vi "CAN_Init-8.6.vi"(0 "CAN卡类型":u32(ring)=4 items=["PCI5121"=1, "PCI9810"=2, "USBCAN1"=3, "USBCAN2"=4, "PCI9820"=5, "PCI5110"=7, "CANLite(mini)"=8, "ISA9620"=9, "ISA5420"=10, "PC104CAN"=11, "DNP9810"=13, "PCI9840B"=14, "PC104C2"=15, "PCI9820I"=16, "pec9920"=18, "USBCAN_E_U"=20, "USBCAN_2E_U"=21], 1 "设备索引号":u16(ring) items=["0", "1", "2", "3", "4", "5", "6", "7", "8", "9", "10", "11", "12", "13", "14", "15", ""], 2 "CAN端口":u16(ring) items=["0", "1"], 3 "波特率":T5(ring)=enum."500Kbps", 4 "操作类型":enum16{"初始化CAN", "关闭CAN"}(ring), 5 "error in (no error)":errorcluster caption="错误输入（无错误）", 6 "滤波方式":u8(ring)=1 items=["Dual Filter", "Single Filter"], 7 "Accept Code":u32 format="%08x", 8 "簇":T3={"打开CAN"=TRUE, "初始化CAN"=TRUE, "开始CAN"=TRUE, "重启"=TRUE, "关闭CAN"=TRUE}, 9 "Mask Code":u32=4294967295 format="%08x", 10 "工作方式":u8(ring) items=["Normal", "Listen Only"], 11 "E-U_baud":u32(ring)=393223 items=["0x060003--1000Kbps"=393219, "0x060004--800Kbps"=393220, "0x060007--500Kbps"=393223, "0x1C0008--250Kbps"=1835016, "0x1C0011--125Kbps"=1835025, "0x160023--100Kbps"=1441827, "0x1C002C--50Kbps"=1835052, "0x1600B3--20Kbps"=1441971, "0x1C00E0--10Kbps"=1835232, "0x1C01C1--5Kbps"=1835457], 12 "是否滤波":bool, 13 "滤波选择":T2={"fiter_mode"=1, "fiter_endid"=0, "fiter_startid"=0} {"fiter_mode" items=["标准帧滤波", "扩展帧滤波", "禁能滤波"]}) -> (14 "CAN 操作结果":bool=TRUE, 18 "真":bool, 19 "error out":errorcluster caption="错误输出")   [LabVIEW 2013]
uses:
  data/ControlCAN.dll
panel:
  out "跳过":bool
  out "数值":u32
  out "VCI_CAN_STATUS 2":T1
  out "ret_ok":bool=TRUE
  out "VCI_FILTER_RECORD":cluster{"ExtFrame":u32, "Start":u32, "End":u32}
  in  "e-u-baud":cluster{"数值":u32}
  in  "VCI_INIT_CONFIG":T4={"AccCode"=0, "AccMask"=4294967295, "Reserved"=0, "Filter"=0, "Timing0"=0, "Timing1"=28, "Mode"=0}
  in  "DeviceType 5":u16(ring)=1 items=["PCI5121"=1, "PCI9810"=2, "USBCAN1"=3, "USBCAN2"=4, "PCI9820"=5, "CAN232"=6, "PCI5110"=7, "CANLite(mini)"=8, "ISA9620"=9, "ISA5420"=10, "PC104CAN"=11, "CANETE"=12, "DNP9810"=13]
  in  "CAN Channel 3":u16(ring) items=["0", "1"]
  in  "DeviceType 4":u16(ring)=1 items=["PCI5121"=1, "PCI9810"=2, "USBCAN1"=3, "USBCAN2"=4, "PCI9820"=5, "CAN232"=6, "PCI5110"=7, "CANLite(mini)"=8, "ISA9620"=9, "ISA5420"=10, "PC104CAN"=11, "CANETE"=12, "DNP9810"=13]
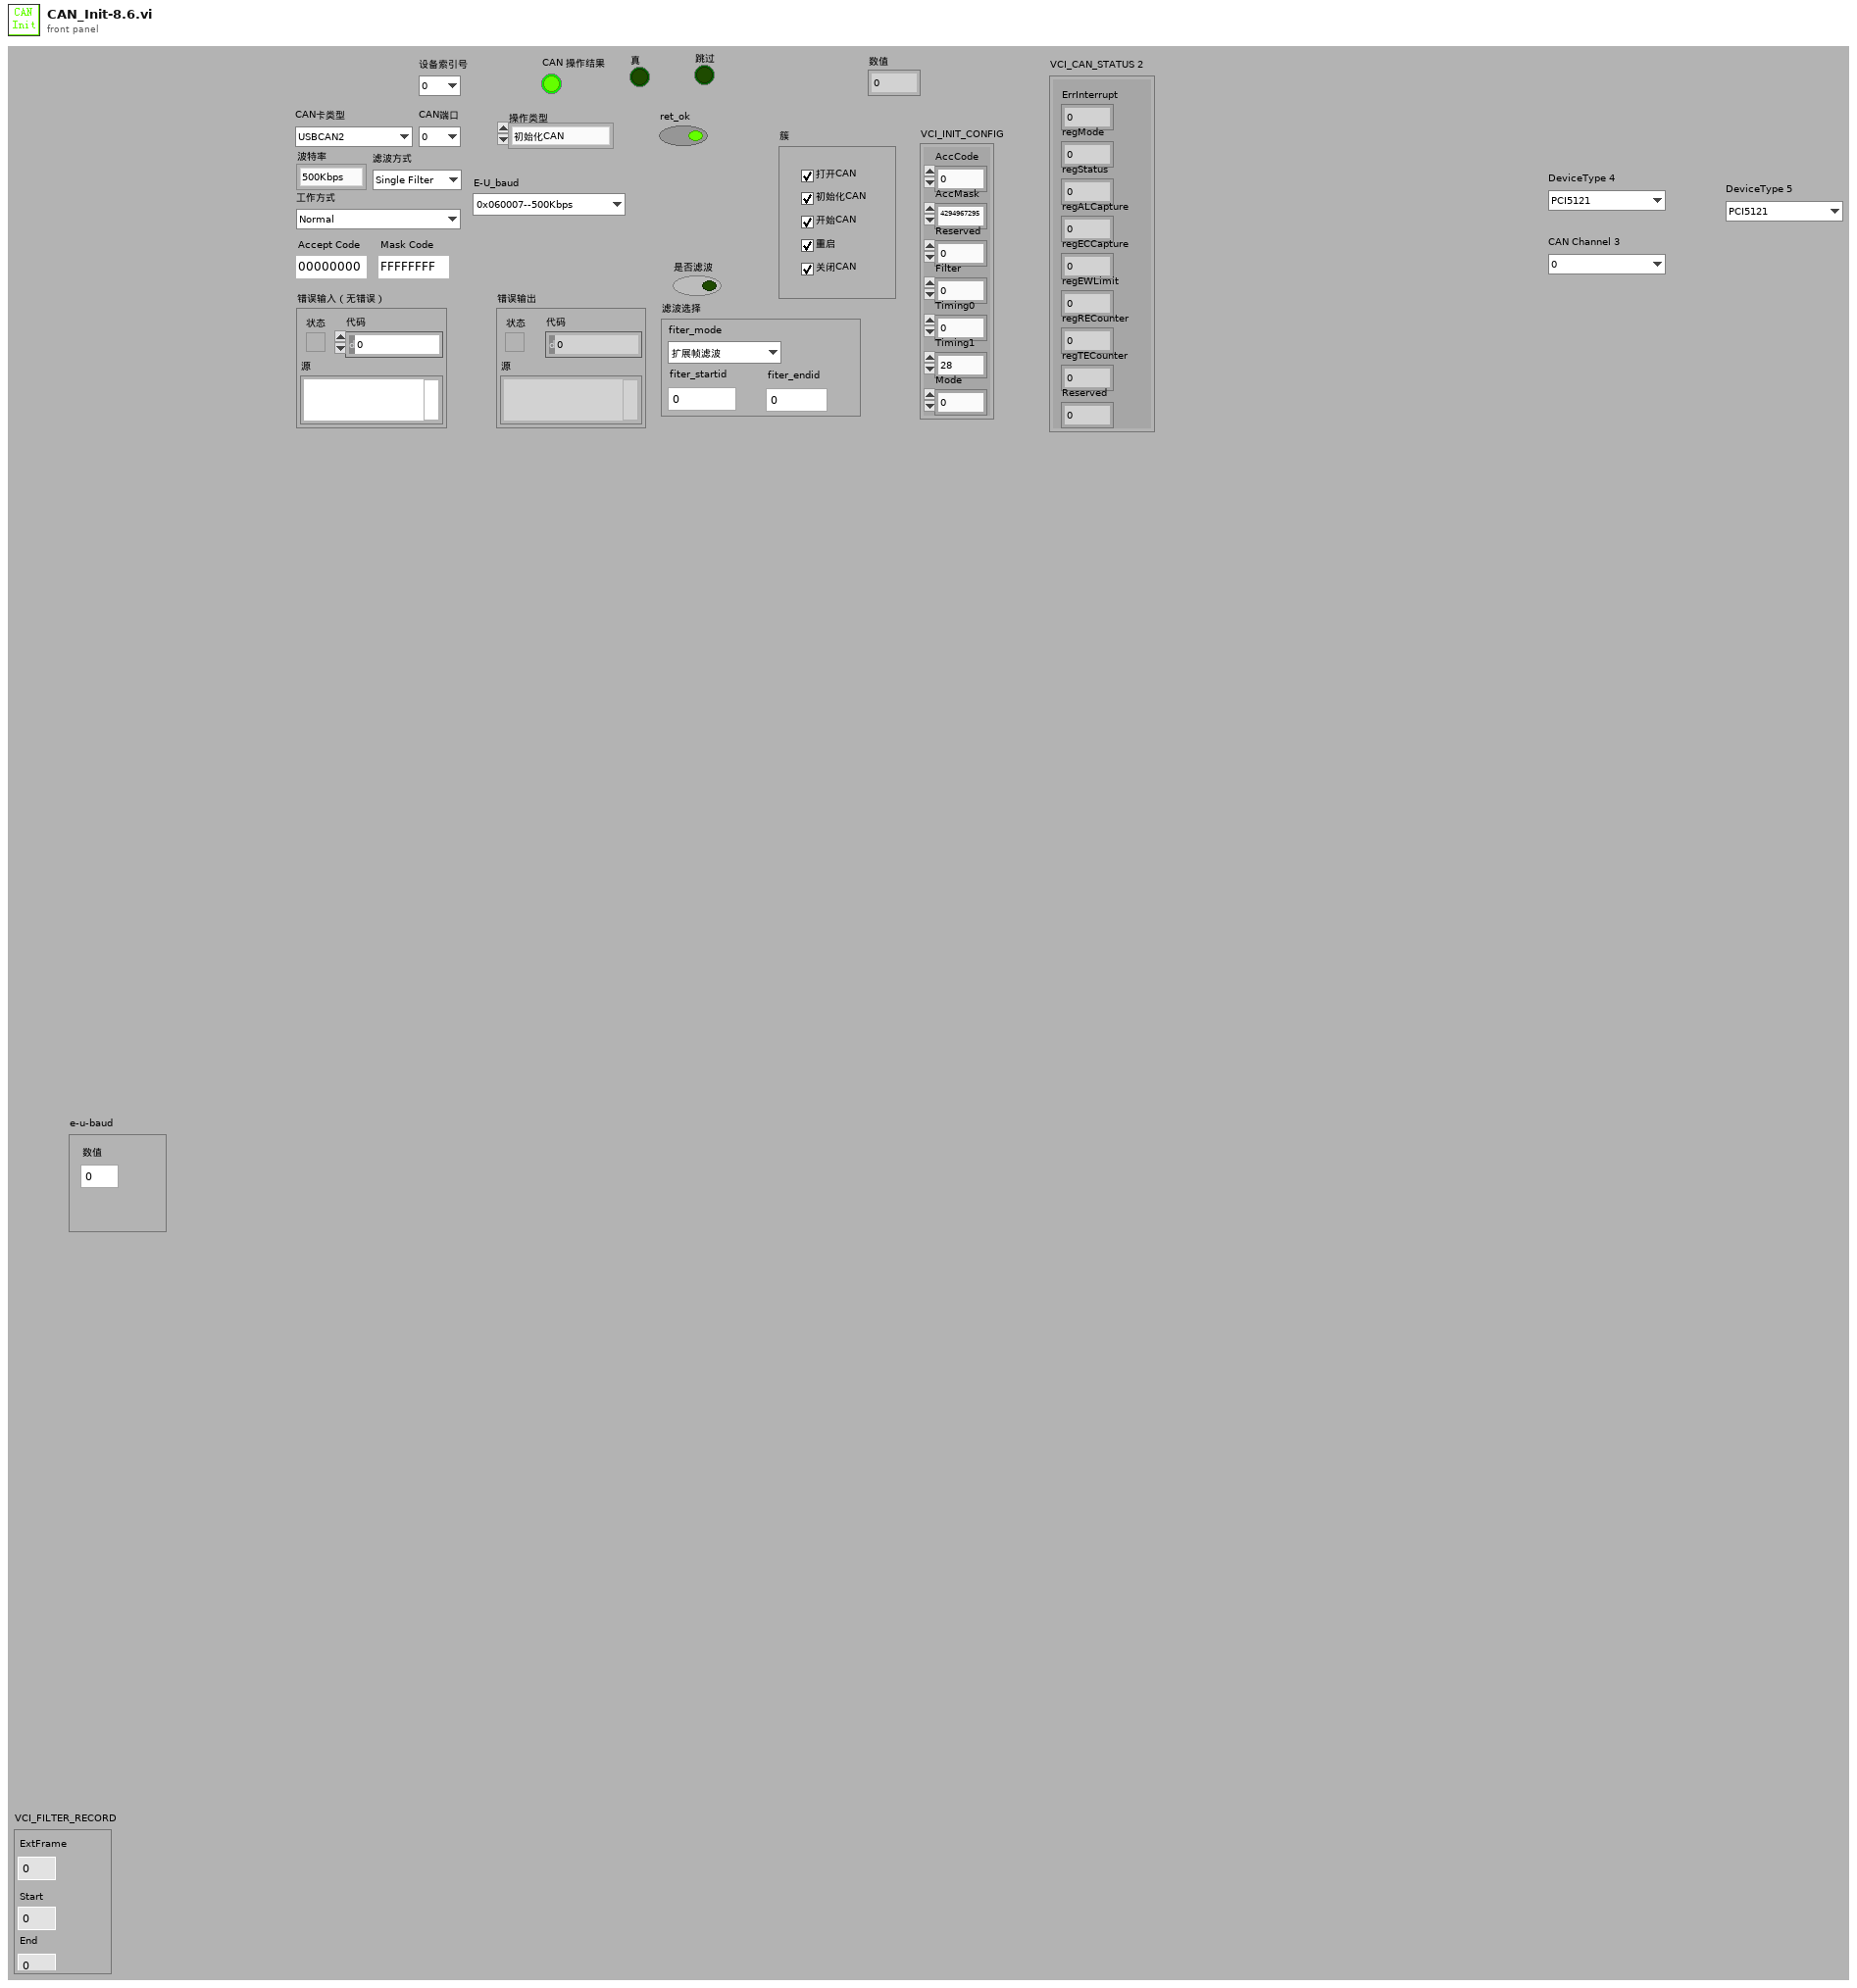
[diagram p1: front panel]
types:
  T1 = cluster{"ErrInterrupt":u8, "regMode":u8, "regStatus":u8, "regALCapture":u8, "regECCapture":u8, "regEWLimit":u8, "regRECounter":u8, "regTECounter":u8, "Reserved":u32}
  T2 = cluster{"fiter_mode":u32, "fiter_endid":u32, "fiter_startid":u32}
  T3 = cluster{"打开CAN":bool, "初始化CAN":bool, "开始CAN":bool, "重启":bool, "关闭CAN":bool}
  T4 = cluster{"AccCode":u32, "AccMask":u32, "Reserved":u32, "Filter":u8, "Timing0":u8, "Timing1":u8, "Mode":u8}
  T5 = enum16{"5Kbps", "10Kbps", "20Kbps", "40Kbps", "50Kbps", "80Kbps", "100Kbps", "125Kbps", "200Kbps", "250Kbps", "400Kbps", "500Kbps", "666Kbps", "800Kbps", "1000Kbps"}
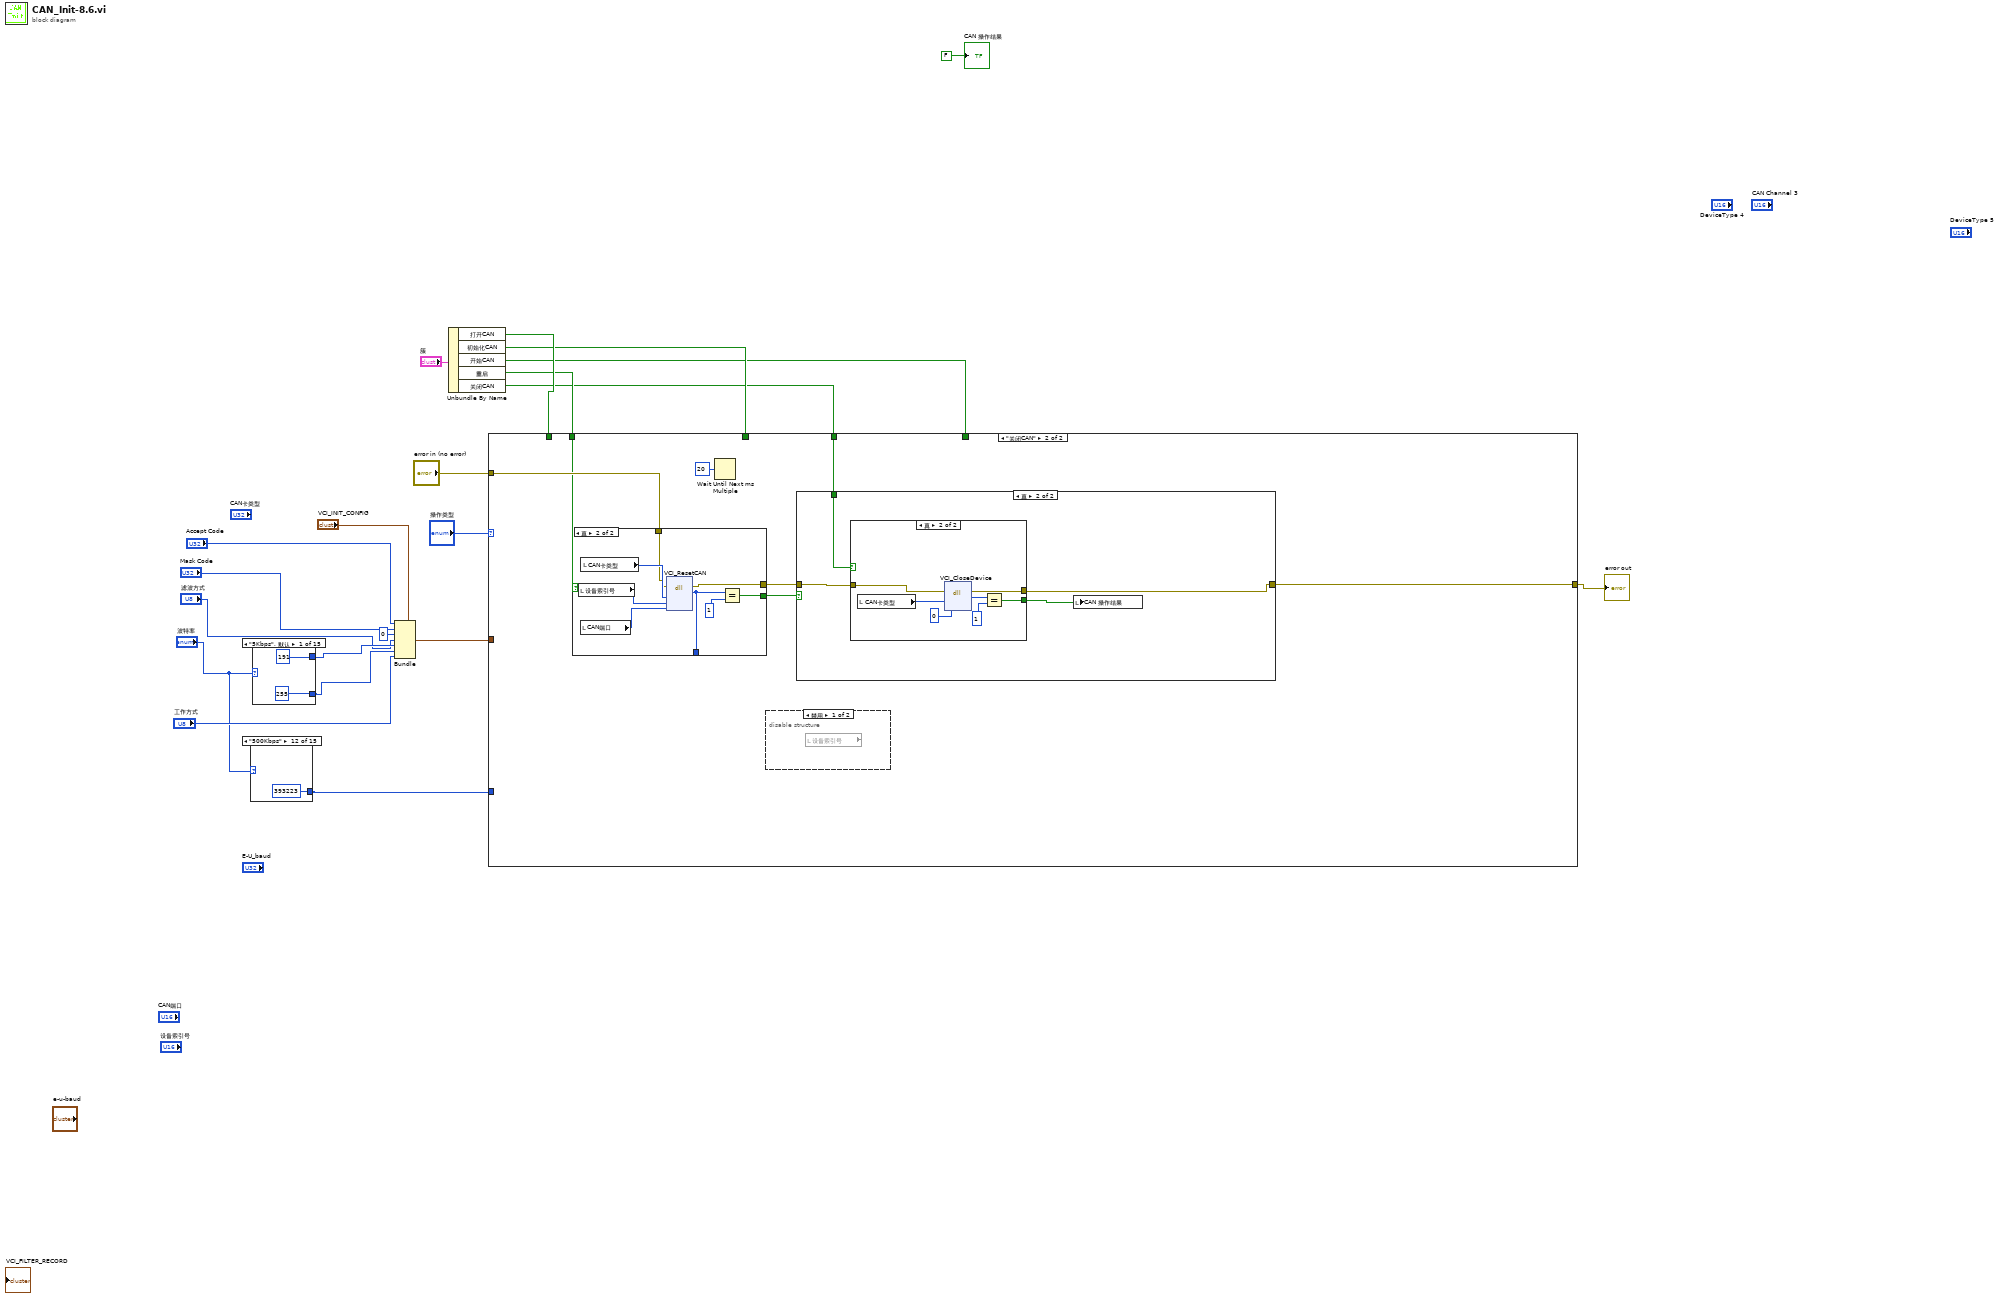
[diagram p0: block diagram]
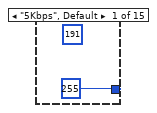
[diagram p2: hidden frame]
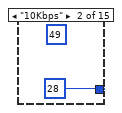
[diagram p3: hidden frame]
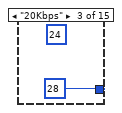
[diagram p4: hidden frame]
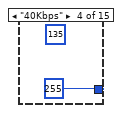
[diagram p5: hidden frame]
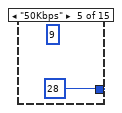
[diagram p6: hidden frame]
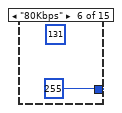
[diagram p7: hidden frame]
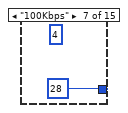
[diagram p8: hidden frame]
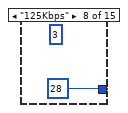
[diagram p9: hidden frame]
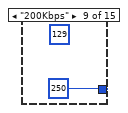
[diagram p10: hidden frame]
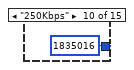
[diagram p11: hidden frame]
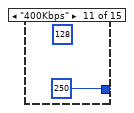
[diagram p12: hidden frame]
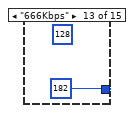
[diagram p13: hidden frame]
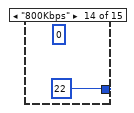
[diagram p14: hidden frame]
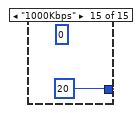
[diagram p15: hidden frame]
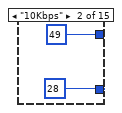
[diagram p16: hidden frame]
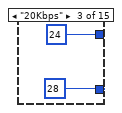
[diagram p17: hidden frame]
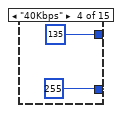
[diagram p18: hidden frame]
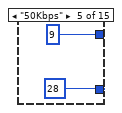
[diagram p19: hidden frame]
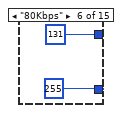
[diagram p20: hidden frame]
diagram:
  n1 = case shown="\"500Kbps\"" "波特率" {
    tunnel: [255 28 28 255 28 255 28 28 250 1835016 250 393223 182 22 20] -> w1
    frame "5Kbps", Default {
      (unwired) 191
    }
    frame "10Kbps" {
      (unwired) 49
    }
    frame "20Kbps" {
      (unwired) 24
    }
    frame "40Kbps" {
      (unwired) 135
    }
    frame "50Kbps" {
      (unwired) 9
    }
    frame "80Kbps" {
      (unwired) 131
    }
    frame "100Kbps" {
      (unwired) 4
    }
    frame "125Kbps" {
      (unwired) 3
    }
    frame "200Kbps" {
      (unwired) 129
    }
    frame "250Kbps" {
    }
    frame "400Kbps" {
      (unwired) 128
    }
    frame "500Kbps" {
    }
    frame "666Kbps" {
      (unwired) 128
    }
    frame "800Kbps" {
      (unwired) 0
    }
    frame "1000Kbps" {
      (unwired) 0
    }
  }
  n2 = case shown="\"5Kbps\", 默认" "波特率" {
    tunnel: [191 49 24 135 9 131 4 3 129 1 128 0 128 0 0] -> w20
    tunnel: [255 28 28 255 28 255 28 28 250 28 250 28 182 22 20] -> w19
    frame "5Kbps", Default {
    }
    frame "10Kbps" {
    }
    frame "20Kbps" {
    }
    frame "40Kbps" {
    }
    frame "50Kbps" {
    }
    frame "80Kbps" {
    }
    frame "100Kbps" {
    }
    frame "125Kbps" {
    }
    frame "200Kbps" {
    }
    frame "250Kbps" {
    }
    frame "400Kbps" {
    }
    frame "500Kbps" {
    }
    frame "666Kbps" {
    }
    frame "800Kbps" {
    }
    frame "1000Kbps" {
    }
  }
  n3 = Bundle(cluster="VCI_INIT_CONFIG", "AccCode"="Accept Code", "AccMask"="Mask Code", "Reserved"=u32 0, "Filter"="滤波方式", "Timing0"=w20, "Timing1"=w19, "Mode"="工作方式") -> (w16:T4)
  n4 = Unbundle By Name("簇") -> ("打开CAN"=w9:bool, "初始化CAN"=w8:bool, "开始CAN"=w7:bool, "重启"=w6:bool, "关闭CAN"=w5:bool)
  n5 = case shown="\"关闭CAN\"" "操作类型" {
    tunnel: w16 -> [w73 _]
    tunnel: "error in (no error)" -> [w72 w242]
    tunnel: [w71 w240] -> w4
    tunnel: w9 -> [w70 _]
    tunnel: w8 -> [w69 _]
    tunnel: w7 -> [w68 _]
    tunnel: w6 -> [_ w239]
    tunnel: w5 -> [_ w238]
    tunnel: w1 -> [w67 _]
    frame "初始化CAN", Default {
      n6 = stacked-sequence {
        seq-local: [w74 _] -> [_ w84]
        tunnel: w73 -> [_ w90]
        tunnel: w72 -> [_ w89]
        tunnel: [_ w88] -> w71
        tunnel: w70 -> [_ w87]
        tunnel: w69 -> [_ w86]
        tunnel: w68 -> [_ w85]
        tunnel: w67 -> [_ w83]
        frame #0 {
          n7 = disable-structure shown="禁用" {
            disable-tunnel: [w75 _] -> w74
            frame Disabled {
              n8 = local read "CAN卡类型"() -> (w81:u32)
              n9 = local read "CAN端口"() -> (w80:u16)
              n10 = dll-call lib="PTH1Fabs EDelan\t上位机BMS_Monitor - 91版_1dataControlCAN.dll" fn="VCI_ReadCANStatus"("DeviceType"=w81, "DeviceInd"=u32 0, "CANInd"=w80) -> ("返回类型"=→"数值":u32, "VCI_CAN_STATUS 2"=w78:T1)  [unwired: 5 in, 4 out]
              "VCI_CAN_STATUS 2" <- w78
              n11 = Unbundle By Name(w78) -> ("regStatus"=w77:u8)
              n12 = Equal?(x=w77, y=u8 18) -> (x = y?=w75:bool)
            }
            frame Enabled {
            }
          }
          "跳过" <- w74
        }
        frame #1 {
          n13 = case shown="假" w84 {
            tunnel: w90 -> [w99 _]
            tunnel: w89 -> [w98 _]
            tunnel: [w96 _] -> w88
            tunnel: w87 -> [w94 _]
            tunnel: w86 -> [w93 _]
            tunnel: w85 -> [w92 _]
            tunnel: w83 -> [w91 _]
            frame False {
              n14 = local read "CAN卡类型"() -> (w95:u32)
              n15 = case shown="真" w94 {
                tunnel: [TRUE w111] -> w101
                tunnel: [w103 w107] -> w100
                tunnel: w98 -> [w105 w110]
                tunnel: [w105 w109] -> w97
                tunnel: [u32 1 ("返回类型") w108] -> _
                tunnel: w95 -> [w103 w107]
                frame False {
                }
                frame True {
                  w106 = 0
                  n16 = dll-call lib="PTH1Fabs EDelan\t上位机BMS_Monitor - 91版_1dataControlCAN.dll" fn="VCI_OpenDevice"(error in=w110, "DevType"=w107, "DevIndex"=w106, "Reserved"=w106) -> (error out=w109:errorcluster, "返回类型"=w108:u32)  [unwired: 4 in, 2 out]
                  n17 = Equal?(x=w108, y=u32 1) -> (x = y?=w111:bool)
                }
              }
              n18 = case shown="真" w101 {
                tunnel: w100 -> [_ w131]
                tunnel: w99 -> [_ w128]
                tunnel: w97 -> [w118 w127]
                tunnel: [w118 w130] -> w96
                tunnel: w93 -> [_ w124]
                tunnel: w92 -> [_ w129]
                tunnel: w91 -> [_ w123]
                frame False {
                  n19 = global read "中英文全局-8.6.vi" "英文?"() -> (w113:bool)
                  n20 = case shown="真" w113 {
                    tunnel: ["Error opening CAN" ("消息") "打开CAN错误" ("消息")] -> w115
                    tunnel: ["Yes" ("按钮名称（“确定”）") "确定" ("按钮名称（“确定”）")] -> w114
                    frame True {
                    }
                    frame False {
                    }
                  }
                  n21 = local write "CAN 操作结果"(FALSE ("初始化结果")) -> ()
                  n22 = One Button Dialog(message=w115, button name ("OK")=w114) -> (true=w116:bool)
                  n23 = local write "真"(w116) -> ()
                }
                frame True {
                  n24 = stacked-sequence {
                    seq-local: [w134 _ _ _] -> [_ w142 _ w193]
                    tunnel: w128 -> [_ _ w171 _]
                    tunnel: [_ _ w170 _] -> _
                    tunnel: w127 -> [_ w141 w169 _]
                    tunnel: [_ _ w168 _] -> w126
                    tunnel: [_ _ w167 _] -> w125
                    tunnel: w124 -> [_ _ w165 _]
                    tunnel: w123 -> [_ w140 _ _]
                    frame #0 {
                      w137 = u32 21 items=["PCI5121"=1, "PCI9810"=2, "USBCAN1"=3, "USBCAN2"=4, "PCI9820"=5, "PCI5110"=7, "CANLite(mini)"=8, "ISA9620"=9, "ISA5420"=10, "PC104CAN"=11, "DNP9810"=13, "PCI9840B"=14, "PC104C2"=15, "PCI9820I"=16, "pec9920"=18, "USBCAN_E_U"=20, "USBCAN_2E_U"=21, ""=0] ("DeviceType")
                      w139 = u32 20 items=["PCI5121"=1, "PCI9810"=2, "USBCAN1"=3, "USBCAN2"=4, "PCI9820"=5, "PCI5110"=7, "CANLite(mini)"=8, "ISA9620"=9, "ISA5420"=10, "PC104CAN"=11, "DNP9810"=13, "PCI9840B"=14, "PC104C2"=15, "PCI9820I"=16, "pec9920"=18, "USBCAN_E_U"=20, "USBCAN_2E_U"=21, ""=0] ("DeviceType")
                      # "判断是不是USB_U_E设备"
                      n25 = local read "CAN卡类型"() -> (w138:u32)
                      n26 = Equal?(x=w138, y=w139) -> (x = y?=w136:bool)
                      n27 = Equal?(x=w138, y=w137) -> (x = y?=w135:bool)
                      n28 = Or(x=w136, y=w135) -> (x .or. y?=w134:bool)
                      n29 = Wait Until Next ms Multiple(millisecond multiple=u32 10 ("毫秒倍数")) -> ()  [unwired: 1 out]
                      "ret_ok" <- TRUE ("ret_ok")
                    }
                    frame #1 {
                      n30 = case shown="真" w142 {
                        tunnel: w141 -> [w143 w148]
                        tunnel: [w143 w147] -> _
                        tunnel: w140 -> [_ w144]
                        frame False {
                          # "不是 -U-E 设备，不做处理"
                        }
                        frame True {
                          # "设置波特率"
                          # "USB-E-U初始化"
                          n31 = local read "CAN卡类型"() -> (w152:u32)
                          n32 = local read "设备索引号"() -> (w151:u16)
                          n33 = local read "CAN端口"() -> (w150:u16)
                          n34 = Bundle(w144) -> (w149:cluster{i32})  [unwired: 1 in]
                          n35 = dll-call lib="PTH1Fabs EDelan\t上位机BMS_Monitor - 91版_1dataControlCAN.dll" fn="VCI_SetReference"(error in=w148, "DevType"=w152, "DevIndex"=w151, "CANInd"=w150, "RefType"=u32 0, "pData"=w149) -> (error out=w147:errorcluster, "返回类型"=w154:u32)  [unwired: 5 in, 3 out]
                          n36 = Wait Until Next ms Multiple(millisecond multiple=u32 10 ("毫秒倍数")) -> ()  [unwired: 1 out]
                          n37 = Equal?(x=w154, y=u32 1) -> (x = y?=w145:bool)
                          n38 = local write "ret_ok"(w145) -> ()
                          n39 = case shown="假" w145 {
                            frame False {
                              n40 = global read "中英文全局-8.6.vi" "英文?"() -> (w156:bool)
                              n41 = case shown="真" w156 {
                                tunnel: ["Set the baud rate error, open the equipment failure" ("消息") "设置波特率错误，打开设备失败" ("消息")] -> w159
                                tunnel: ["Yes" ("按钮名称（“确定”）") "Yes" ("按钮名称（“确定”）")] -> w158
                                frame True {
                                }
                                frame False {
                                }
                              }
                              n42 = One Button Dialog(message=w159, button name ("OK")=w158) -> (true=w157:bool)
                              n43 = local write "真"(w157) -> ()
                            }
                            frame True {
                            }
                          }
                        }
                      }
                    }
                    frame #2 {
                      n44 = local read "ret_ok"() -> (w164:bool)
                      n45 = And(x=w164, y=w165) -> (x .and. y?=w166:bool)
                      n46 = case shown="真" w166 {
                        tunnel: w171 -> [_ w178]
                        tunnel: [_ w177] -> w170
                        tunnel: w169 -> [w172 w176]
                        tunnel: [w172 w175] -> w168
                        tunnel: [_ w174] -> w167
                        tunnel: w164 -> [_ _]
                        frame False {
                        }
                        frame True {
                          n47 = local read "CAN卡类型"() -> (w181:u32)
                          n48 = local read "设备索引号"() -> (w180:u16)
                          n49 = local read "CAN端口"() -> (w179:u16)
                          n50 = dll-call lib="PTH1Fabs EDelan\t上位机BMS_Monitor - 91版_1dataControlCAN.dll" fn="VCI_InitCAN"(error in=w176, "DeviceType"=w181, "DeviceInd"=w180, "CANInd"=w179, "pInitConfig"=w178) -> (error out=w175:errorcluster, "返回类型"=w177:u32)  [unwired: 4 in, 3 out]
                          n51 = Equal?(x=w177, y=u32 1) -> (x = y?=w174:bool)
                          n52 = case shown="假" w174 {
                            frame False {
                              n53 = global read "中英文全局-8.6.vi" "英文?"() -> (w183:bool)
                              n54 = case shown="真" w183 {
                                tunnel: ["Init error" ("消息") "初始化错误" ("消息")] -> w186
                                tunnel: ["Yes" ("按钮名称（“确定”）") "确定" ("按钮名称（“确定”）")] -> w185
                                frame True {
                                }
                                frame False {
                                }
                              }
                              n55 = One Button Dialog(message=w186, button name ("OK")=w185) -> (true=→"真":bool)
                            }
                            frame True {
                            }
                          }
                          n56 = local write "ret_ok"(w174) -> ()
                          n57 = Wait Until Next ms Multiple(millisecond multiple=u32 10 ("毫秒倍数")) -> ()  [unwired: 1 out]
                        }
                      }
                    }
                    frame #3 {
                      n58 = local read "ret_ok"() -> (w192:bool)
                      n59 = And(x=w193, y=w192) -> (x .and. y?=w194:bool)
                      n60 = case shown="真" w194 {
                        frame False {
                        }
                        frame True {
                          n61 = case shown="真" "是否滤波" {
                            frame False {
                            }
                            frame True {
                              w199 = u32 2 items=["标准帧滤波", "扩展帧滤波", "禁能滤波"] ("fiter_mode")
                              # "设置波特率正确，就设置滤波"
                              n62 = local read "滤波选择"() -> (w197:T2)
                              n63 = Unbundle By Name(w197) -> ("fiter_mode"=w196:u32)
                              n64 = Not Equal?(x=w196, y=w199) -> (x != y?=w198:bool)
                              n65 = case shown="真" w198 {
                                frame False {
                                }
                                frame True {
                                n66 = stacked-sequence {
                                frame #0 {
                                n67 = local read "CAN卡类型"() -> (w203:u32)
                                n68 = local read "设备索引号"() -> (w202:u16)
                                n69 = local read "CAN端口"() -> (w201:u16)
                                n70 = dll-call lib="PTH1Fabs EDelan\t上位机BMS_Monitor - 91版_1dataControlCAN.dll" fn="VCI_SetReference"("DevType"=w203, "DevIndex"=w202, "CANInd"=w201, "RefType"=u32 1, "pData"="滤波选择") -> ()  [unwired: 6 in, 5 out]
                                }
                                frame #1 {
                                n71 = local read "CAN卡类型"() -> (w208:u32)
                                n72 = local read "设备索引号"() -> (w207:u16)
                                n73 = local read "CAN端口"() -> (w206:u16)
                                n74 = dll-call lib="PTH1Fabs EDelan\t上位机BMS_Monitor - 91版_1dataControlCAN.dll" fn="VCI_SetReference"("DevType"=w208, "DevIndex"=w207, "CANInd"=w206, "RefType"=u32 2, "pData"=u32 0 ("RefType")) -> ("返回类型"=w210:u32)  [unwired: 5 in, 5 out]
                                n75 = Equal?(x=w210, y=u32 1) -> (x = y?=w205:bool)
                                n76 = case shown="假" w205 {
                                frame False {
                                n77 = global read "中英文全局-8.6.vi" "英文?"() -> (w213:bool)
                                n78 = case shown="假" w213 {
                                tunnel: ["Set the filter failure!" ("消息") "设置滤波失败!" ("消息")] -> w215
                                tunnel: ["Yes" ("按钮名称（“确定”）") "是" ("按钮名称（“确定”）")] -> w214
                                frame True {
                                }
                                frame False {
                                }
                                }
                                n79 = One Button Dialog(message=w215, button name ("OK")=w214) -> ()  [unwired: 1 out]
                                }
                                frame True {
                                }
                                }
                                n80 = local write "ret_ok"(w205) -> ()
                                }
                                }
                                }
                              }
                            }
                          }
                        }
                      }
                      n81 = Wait Until Next ms Multiple(millisecond multiple=u32 10 ("毫秒倍数")) -> ()  [unwired: 1 out]
                    }
                  }
                  n82 = case shown="真" w125 {
                    tunnel: w131 -> [_ w226]
                    tunnel: w126 -> [w220 w224]
                    tunnel: [w220 w223] -> w130
                    tunnel: w129 -> [_ w222]
                    frame False {
                      n83 = local write "CAN 操作结果"(FALSE ("初始化结果")) -> ()
                    }
                    frame True {
                      n84 = case shown="真" w222 {
                        tunnel: w226 -> [_ w234]
                        tunnel: [FALSE w231] -> w225
                        tunnel: w224 -> [w227 w230]
                        tunnel: [w227 w229] -> w223
                        frame False {
                        }
                        frame True {
                          n85 = local read "设备索引号"() -> (w233:u16)
                          n86 = local read "CAN端口"() -> (w232:u16)
                          n87 = dll-call lib="PTH1Fabs EDelan\t上位机BMS_Monitor - 91版_1dataControlCAN.dll" fn="VCI_StartCAN"(error in=w230, "DeviceType"=w234, "DeviceInd"=w233, "CANInd"=w232) -> (error out=w229:errorcluster, "返回类型"=w235:u32)  [unwired: 3 in, 3 out]
                          n88 = Equal?(x=w235, y=u32 1) -> (x = y?=w231:bool)
                        }
                      }
                      n89 = local write "CAN 操作结果"(w225) -> ()
                    }
                  }
                }
              }
            }
            frame True {
            }
          }
        }
      }
    }
    frame "关闭CAN" {
      n90 = case shown="真" w239 {
        tunnel: [TRUE w254] -> w243
        tunnel: w242 -> [w247 w250]
        tunnel: [w247 w249] -> w241
        tunnel: [u32 1 ("返回类型") w248] -> _
        frame False {
          n91 = Wait Until Next ms Multiple(millisecond multiple=u32 10 ("毫秒倍数")) -> ()  [unwired: 1 out]
        }
        frame True {
          n92 = local read "设备索引号"() -> (w252:u16)
          n93 = local read "CAN端口"() -> (w251:u16)
          n94 = local read "CAN卡类型"() -> (w253:u32)
          n95 = dll-call lib="PTH1Fabs EDelan\t上位机BMS_Monitor - 91版_1dataControlCAN.dll" fn="VCI_ResetCAN"(error in=w250, "DeviceType"=w253, "DeviceInd"=w252, "CANInd"=w251) -> (error out=w249:errorcluster, "返回类型"=w248:u32)  [unwired: 3 in, 3 out]
          n96 = Equal?(x=w248, y=u32 1) -> (x = y?=w254:bool)
        }
      }
      n97 = Wait Until Next ms Multiple(millisecond multiple=u32 20 ("毫秒倍数")) -> ()  [unwired: 1 out]
      n98 = disable-structure shown="禁用" {
        frame Disabled {
          n99 = local read "设备索引号"() -> ()  [unwired: 1 out]
        }
        frame Enabled {
        }
      }
      n100 = case shown="真" w243 {
        tunnel: w241 -> [w256 w261]
        tunnel: [w256 w260] -> w240
        tunnel: w238 -> [_ w259]
        frame False {
          n101 = local write "CAN 操作结果"(FALSE ("CAN 操作结果")) -> ()
        }
        frame True {
          n102 = case shown="真" w259 {
            tunnel: [FALSE w268] -> w258
            tunnel: w261 -> [w262 w267]
            tunnel: [w262 w266] -> w260
            frame False {
            }
            frame True {
              n103 = local read "CAN卡类型"() -> (w269:u32)
              n104 = dll-call lib="PTH1Fabs EDelan\t上位机BMS_Monitor - 91版_1dataControlCAN.dll" fn="VCI_CloseDevice"(error in=w267, "DeviceType"=w269, "DeviceInd"=u32 0) -> (error out=w266:errorcluster, "返回类型"=w265:u32)  [unwired: 3 in, 2 out]
              n105 = Equal?(x=w265, y=u32 1) -> (x = y?=w268:bool)
            }
          }
          n106 = local write "CAN 操作结果"(w258) -> ()
        }
      }
    }
  }
  "error out" <- w4
  "CAN 操作结果" <- FALSE ("CAN 操作结果")
